vi "MagRetBypass_Global.vi"() -> ()   [LabVIEW 2019]
panel:
  out "MRB_ST":u32(colorbox)
  out "MRB_opening":dbl
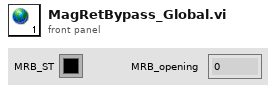
[diagram p1: front panel]
diagram:
